vi "Read Parameter (Now).vi"(8 "error in (no error)":errorcluster, 11 "SweepControl in":refnum<class "SweepControl.lvclass">) -> (0 "error out":errorcluster, 2 "Parameter (Now)":dbl, 3 "SweepControl out":refnum<class "SweepControl.lvclass">)   [LabVIEW 2016, in "SweepControl.lvclass"]
uses:
  SweepControl.lvclass
  SweepControl.lvclass/SweepControl.ctl
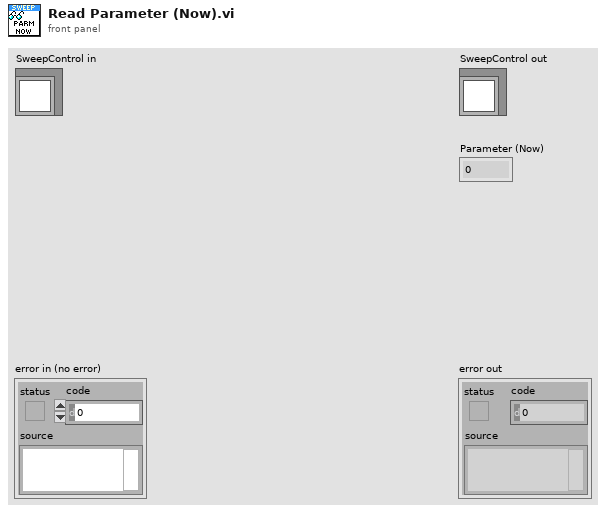
[diagram p1: front panel]
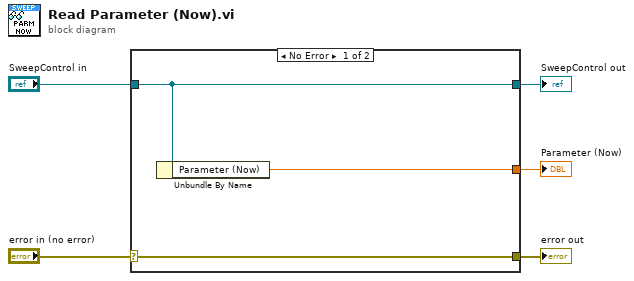
[diagram p0: block diagram]
diagram:
  n1 = case shown="No Error" "error in (no error)" {
    selector: "error in (no error)" -> [w8 w9]
    tunnel: [w8 w9] -> w4
    tunnel: [w7 w10] -> w2
    tunnel: "SweepControl in" -> [w7 w10]
    tunnel: [w6 _] -> w1
    frame No Error {
      n2 = Unbundle By Name(w7) -> ("Parameter (Now)"=w6:dbl)
    }
    frame Error {
    }
  }
  "error out" <- w4
  "SweepControl out" <- w2
  "Parameter (Now)" <- w1
